vi "Execute VI Action.vi"(8 "Error In":errorcluster, 10 "VI":path, 11 "Menu Tag":string) -> (0 "Error Out":errorcluster)   [LabVIEW 2018, in "Bookmark Manager.lvlib"]
uses:
  Bookmark Manager.lvlib
  Toolkit/Toolkit.lvlib
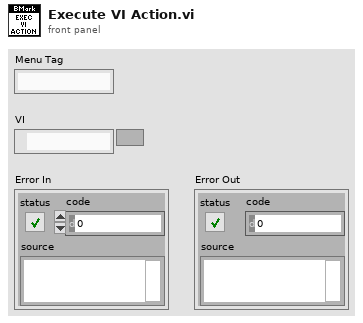
[diagram p1: front panel]
types:
  T1 = enum32{"Bad", "Idle", "Run top level", "Running"}
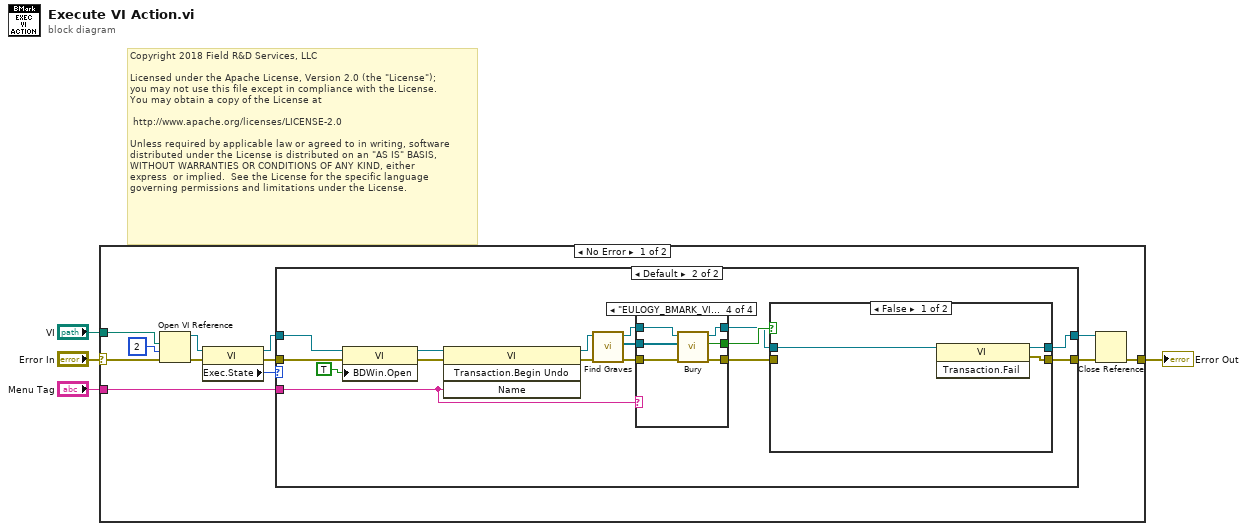
[diagram p0: block diagram]
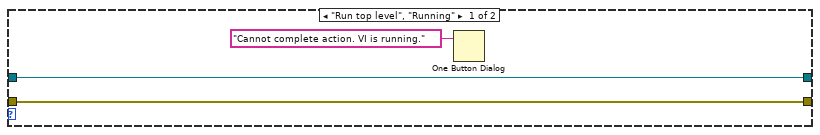
[diagram p2: hidden frame]
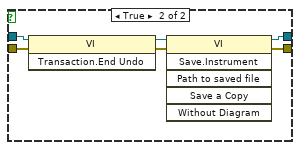
[diagram p3: hidden frame]
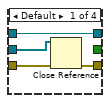
[diagram p4: hidden frame]
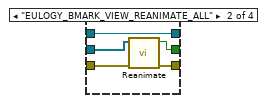
[diagram p5: hidden frame]
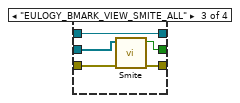
[diagram p6: hidden frame]
diagram:
  # "Copyright 2018 Field R&D Services, LLC\n\nLicensed under the Apache License, Version 2.0 (the \"License\");\nyou may not use this file except in compliance with the License.\nYou may obtain a copy of the License at\n\n\thttp://www.apache.org/licenses/LICENSE-2.0\n\nUnless required by applicable law or agreed to in writing, software\ndistributed under the License is distributed on an \"AS IS\" BASIS,\nWITHOUT WARRANTIES OR CONDITIONS OF ANY KIND, either \nexpress  or implied.  See the License for the specific language \ngoverning permissions and limitations under the License."
  n1 = case shown="No Error" "Error In" {
    selector: "Error In" -> [w6 w65]
    tunnel: [w16 w65] -> w4
    tunnel: "Menu Tag" -> [w15 _]
    tunnel: "VI" -> [w5 _]
    frame No Error {
      n2 = Open VI Reference(vi path=w5, options=2, error in (no error)=w6) -> (vi reference=w9:refnum<vi>, error out=w8:errorcluster)  [unwired: 3 in]
      n3 = property class="VI"(reference=w9, error in=w8) -> (reference out=w12:refnum<vi>, error out=w13:errorcluster, "Exec.State"=w14:T1)
      n4 = case shown="Default" w14 {
        tunnel: [w18 w29] -> w10
        tunnel: w13 -> [w18 w35]
        tunnel: w12 -> [w19 w34]
        tunnel: [w19 w30] -> w11
        tunnel: w15 -> [_ w26]
        frame "Run top level", "Running" {
          n5 = One Button Dialog(message="Cannot complete action. VI is running.") -> ()  [unwired: 1 in, 1 out]
        }
        frame Default {
          n6 = property class="VI"(reference=w34, error in=w35, "BDWin.Open"=TRUE ("Block Diagram Window:Open")) -> (reference out=w33:refnum<vi>, error out=w32:errorcluster)
          n7 = invoke class="VI" method="Transaction.Begin Undo"(reference=w33, error in=w32, "Name"=w26) -> (reference out=w22:refnum<vi>, error out=w24:errorcluster)  [unwired: 1 in, 2 out]
          n8 = call "Find Graves.vi"("Error In"=w24, "VI In"=w22) -> ("Error Out"=w23:errorcluster, "Graves"=w25:refnum<vi>[], "VI Out"=w21:refnum<vi>)  [unwired: 7 in]
          n9 = case shown="\"EULOGY_BMARK_VIEW_BURY_ALL\"" w26 {
            tunnel: [w47 w53 w57 w64] -> w28
            tunnel: [_ w52 w56 w62] -> w27
            tunnel: w23 -> [w48 w51 w58 w63]
            tunnel: w25 -> [w46 w50 w55 w59]
            tunnel: w21 -> [w45 w49 w54 w61]
            tunnel: [w45 w49 w54 w60] -> w20
            frame Default {
              n10 = Close Reference(reference=w46, error in (no error)=w48) -> (error out=w47:errorcluster)
            }
            frame "EULOGY_BMARK_VIEW_REANIMATE_ALL" {
              n11 = call "Reanimate.vi"("Error In"=w51, "Graves"=w50) -> ("Error Out"=w53:errorcluster, "Change Made?"=w52:bool)  [unwired: 8 in]
            }
            frame "EULOGY_BMARK_VIEW_SMITE_ALL" {
              n12 = call "Smite.vi"("Error In"=w58, "Graves"=w55) -> ("Error Out"=w57:errorcluster, "Change Made?"=w56:bool)  [unwired: 8 in]
            }
            frame "EULOGY_BMARK_VIEW_BURY_ALL" {
              n13 = call "Bury.vi"("Error In"=w63, "Graves"=w59, "VI In"=w61) -> ("Error Out"=w64:errorcluster, "Change Made?"=w62:bool, "VI Out"=w60:refnum<vi>)  [unwired: 6 in]
            }
          }
          n14 = case shown="False" w27 {
            tunnel: [w38 w43] -> w30
            tunnel: [w37 w41] -> w29
            tunnel: w28 -> [_ w40]
            tunnel: w20 -> [w36 w39]
            frame False {
              n15 = invoke class="VI" method="Transaction.Fail"(reference=w36) -> (reference out=w38:refnum<vi>, error out=w37:errorcluster)  [unwired: 2 in, 1 out]
            }
            frame True {
              n16 = invoke class="VI" method="Transaction.End Undo"(reference=w39, error in=w40) -> (reference out=w44:refnum<vi>, error out=w42:errorcluster)  [unwired: 1 in, 1 out]
              n17 = invoke class="VI" method="Save.Instrument"(reference=w44, error in=w42) -> (reference out=w43:refnum<vi>, error out=w41:errorcluster)  [unwired: 4 in, 4 out]
            }
          }
        }
      }
      n18 = Close Reference(reference=w11, error in (no error)=w10) -> (error out=w16:errorcluster)
    }
    frame Error {
    }
  }
  "Error Out" <- w4
